vi "Make output waveforms.vi"(4 "after":dbl, 6 "before":dbl, 9 "dt":dbl, 10 "stimphases in":T2, 11 "output":dbl[](array[numeric])) -> (2 "stimphases out":T1, 3 "output waveform":waveform(dbl))   [LabVIEW 2013]
uses:
  Stim phases.ctl
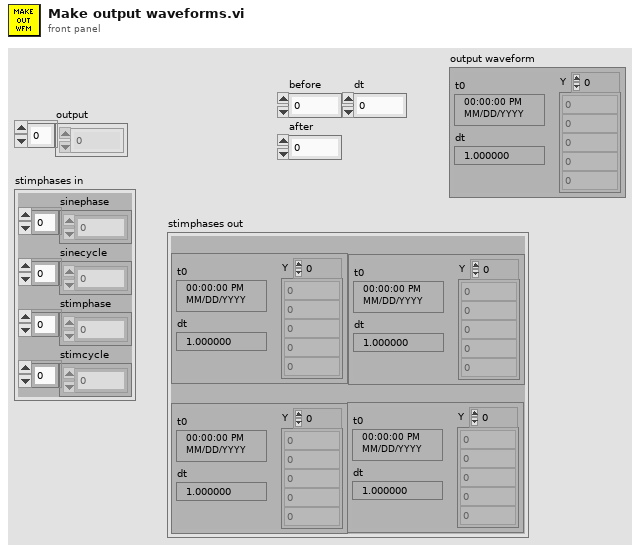
[diagram p1: front panel]
types:
  T1 = typedef "Stim phases.ctl" = cluster{"sinephase":waveform(dbl), "sinecycles":waveform(dbl), "stimphase":waveform(dbl), "stimcycles":waveform(dbl)}
  T2 = cluster{"sinephase":dbl[], "sinecycle":dbl[], "stimphase":dbl[], "stimcycle":dbl[]}
  T3 = cluster{waveform(dbl), waveform(dbl), waveform(dbl), waveform(dbl)}
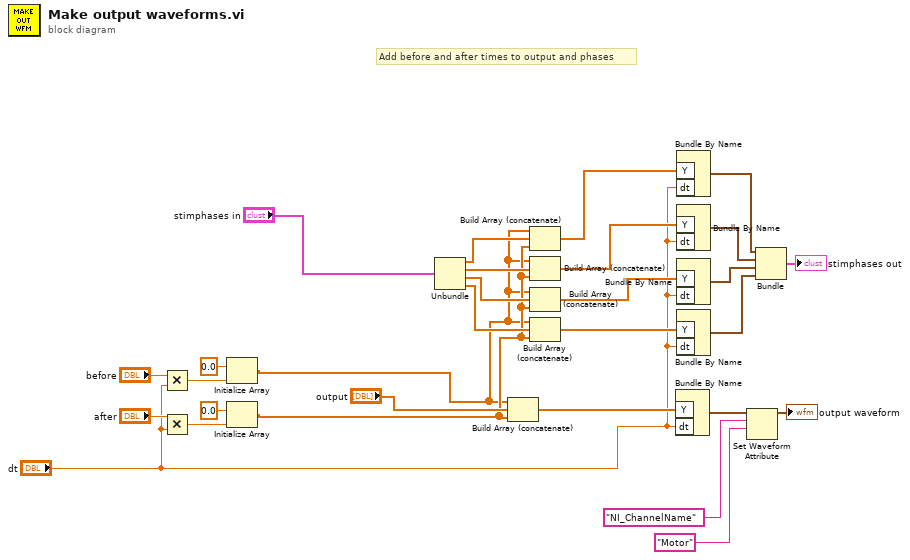
[diagram p0: block diagram]
diagram:
  # "Add before and after times to output and phases"
  n1 = Multiply(x="before", y="dt") -> (x*y=w22:dbl)
  n2 = Multiply(x="after", y="dt") -> (x*y=w20:dbl)
  n3 = Initialize Array(0.0 ("element"), w22) -> (w16:dbl[])
  n4 = Initialize Array(0.0 ("element"), w20) -> (w17:dbl[])
  n5 = Unbundle("stimphases in") -> ("sinephase"=w25:dbl[], "sinecycle"=w26:dbl[], "stimphase"=w27:dbl[], "stimcycle"=w28:dbl[])
  n6 = Build Array (concatenate)(w16, "output", w17) -> (w15:dbl[])
  n7 = Build Array (concatenate)(w16, w25, w17) -> (w11:dbl[])
  n8 = Build Array (concatenate)(w16, w26, w17) -> (w10:dbl[])
  n9 = Build Array (concatenate)(w16, w27, w17) -> (w9:dbl[])
  n10 = Build Array (concatenate)(w16, w28, w17) -> (w8:dbl[])
  n11 = Bundle By Name("Y"=w15, "dt"="dt") -> (w14:waveform(dbl))  [unwired: 1 in]
  n12 = Bundle By Name("Y"=w11, "dt"="dt") -> (w6:waveform(dbl))  [unwired: 1 in]
  n13 = Bundle By Name("Y"=w10, "dt"="dt") -> (w5:waveform(dbl))  [unwired: 1 in]
  n14 = Bundle By Name("Y"=w9, "dt"="dt") -> (w4:waveform(dbl))  [unwired: 1 in]
  n15 = Bundle By Name("Y"=w8, "dt"="dt") -> (w3:waveform(dbl))  [unwired: 1 in]
  n16 = Set Waveform Attribute(5:"Motor" ("name"), 6:"NI_ChannelName" ("name"), 7:w14) -> (3:→"output waveform":waveform(dbl))  [unwired: 1 in, 2 out]
  n17 = Bundle(w6, w5, w4, w3) -> (→"stimphases out":T3)  [unwired: 1 in]
